vi "Trans.vi"   [LabVIEW 2013, in "标准状态机模板.lvlib"]
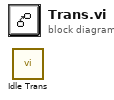
[diagram p0: block diagram]
diagram:
  n1 = call "Idle Trans.vi"() -> ()  [unwired: 9 in, 3 out]
